vi "MALT Get Devices.vi"(8 "error in":errorcluster) -> (0 "error out":errorcluster, 3 "Devices":string[](array[string]))   [LabVIEW 2018]
panel:
  out "Response":string
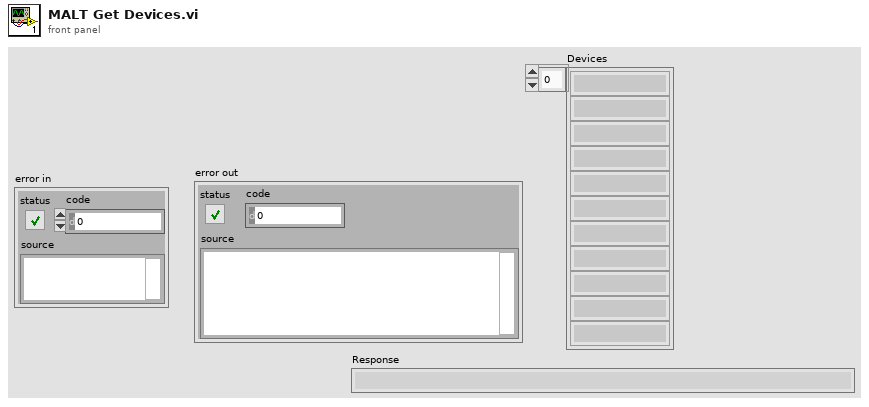
[diagram p1: front panel]
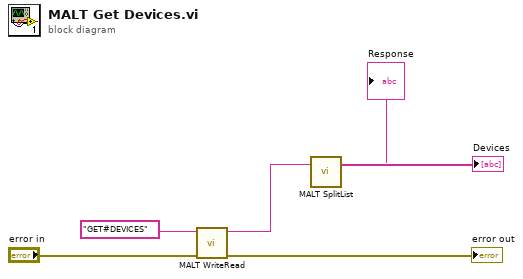
[diagram p0: block diagram]
diagram:
  n1 = call "MALT WriteRead.vi"("error in"="error in", "Request"="GET#DEVICES" ("data in")) -> ("error out"=→"error out":errorcluster, "Response"=w1:string)  [unwired: 8 in]
  "Response" <- w1
  n2 = call "MALT SplitList.vi"("Line"=w1) -> ("Items"=→"Devices":string[])  [unwired: 2 in]
